vi "output_steps_slower.vi"(7 "# of Samples":i32=7000, 9 "Offset / V":cluster{"X":dbl, "Y":dbl, "Z":dbl}={"X"=0.0, "Y"=0.0, "Z"=0.5}, 10 "Amplitude / V":dbl=0.1 format="%.2g") -> (2 "Output":dbl[][](graph))   [LabVIEW 2018]
panel:
  # "This code is not very adjustable. The number \nof substeps cannot be changed without causing it\nto go haywire and is fixed at 10.\nThe substeps are 300 samples long; 250 as still and \n50 slewing"
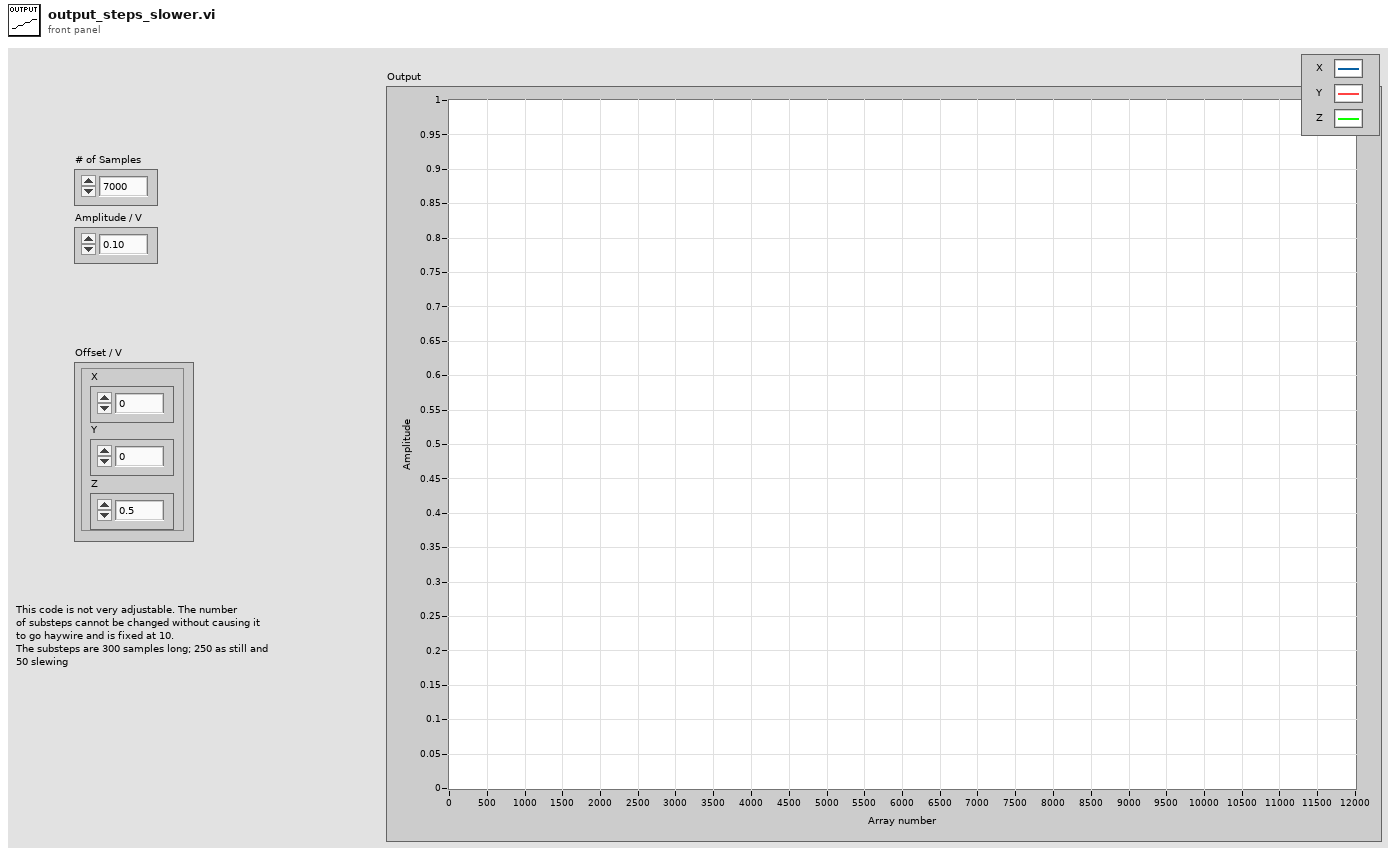
[diagram p1: front panel]
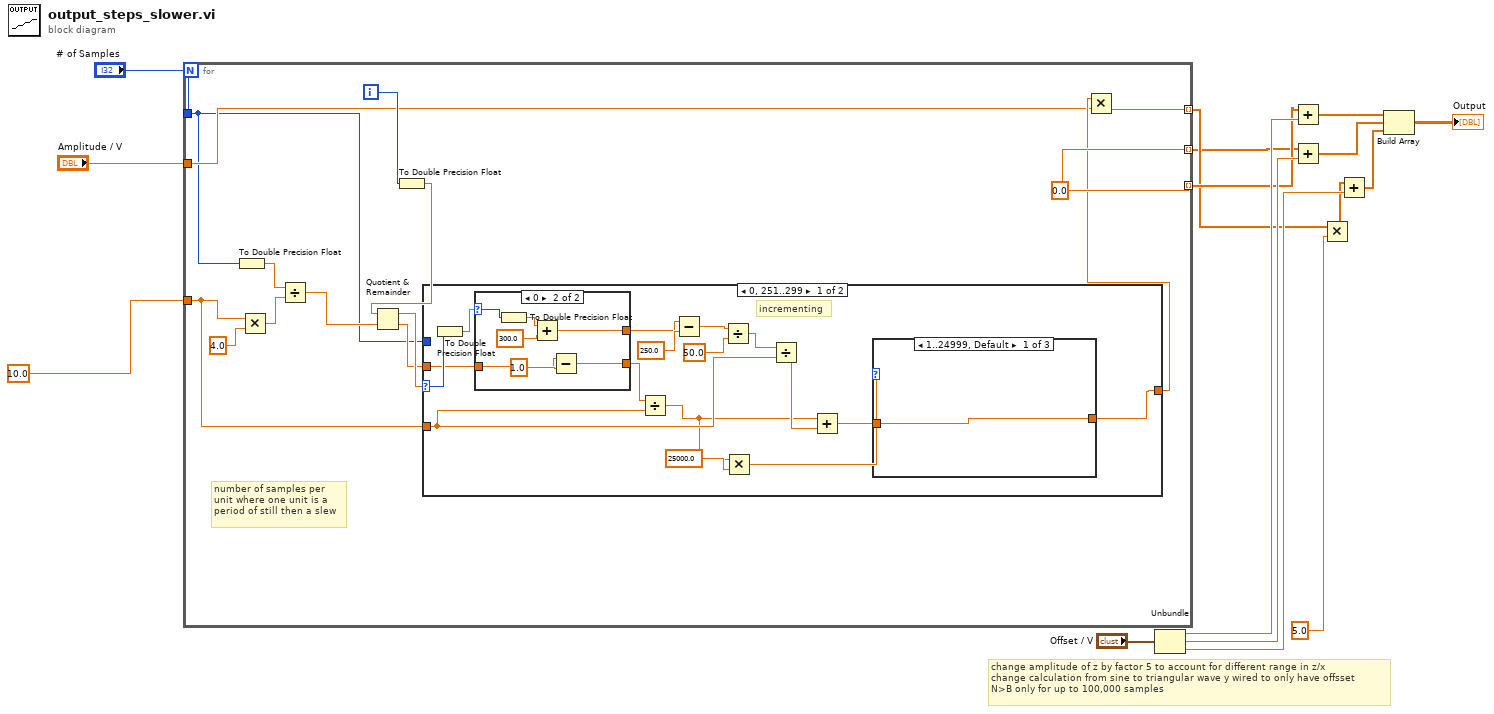
[diagram p0: block diagram]
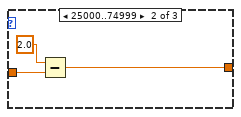
[diagram p3: hidden frame]
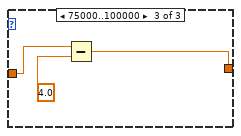
[diagram p4: hidden frame]
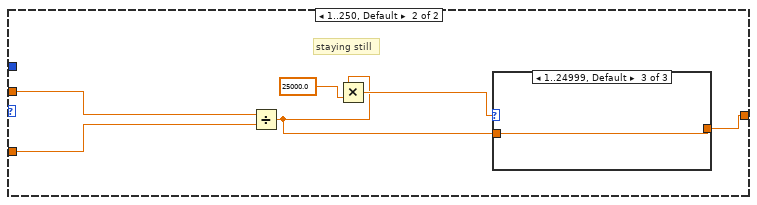
[diagram p5: hidden frame]
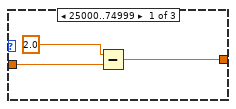
[diagram p6: hidden frame]
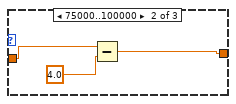
[diagram p7: hidden frame]
diagram:
  # "change amplitude of z by factor 5 to account for different range in z/x\nchange calculation from sine to triangular wave y wired to only have offsset\nN>B only for up to 100,000 samples"
  n1 = for {
    N: "# of Samples" -> [_]
    tunnel: [w30] -> w5 mode=indexing
    tunnel: [w29] -> w2 mode=indexing
    tunnel: "# of Samples" -> [w19]
    tunnel: "Amplitude / V" -> [w20]
    tunnel: [w29] -> w6 mode=indexing
    tunnel: 10.0 ("number of substeps\nin each direction") -> [w17]
    i -> [w22]
    w29 = 0.0
    # "number of samples per \nunit where one unit is a \nperiod of still then a slew"
    n2 = To Double Precision Float(number=w19) -> (double precision float=w27:dbl)
    n3 = Multiply(x=w17, y=4.0) -> (x*y=w18:dbl)
    n4 = Divide(x=w27, y=w18) -> (x/y=w26:dbl)
    n5 = To Double Precision Float(number=w22) -> (double precision float=w21:dbl)
    n6 = Quotient & Remainder(x=w21, y=w26) -> (x-y*floor(x/y)=w25:dbl, floor(x/y)=w24:dbl)
    n7 = case shown="0, 251..299" w25 {
      selector: w25 -> [w35 _]
      tunnel: w24 -> [w32 w68]
      tunnel: w17 -> [w39 w67]
      tunnel: [w46 w64] -> w23
      tunnel: w19 -> [_ _]
      frame 0, 251..299 {
        # "incrementing"
        n8 = To Double Precision Float(number=w35) -> (double precision float=w33:dbl)
        n9 = case shown="0" w33 {
          selector: w33 -> [w48 w53]
          tunnel: [w48 w54] -> w34
          tunnel: w32 -> [w47 w50]
          tunnel: [w47 w49] -> w31
          frame 251..299, Default {
          }
          frame 0 {
            n10 = To Double Precision Float(number=w53) -> (double precision float=w52:dbl)
            n11 = Add(x=w52, y=300.0) -> (x+y=w54:dbl)
            n12 = Subtract(x=w50, y=1.0) -> (x-y=w49:dbl)
          }
        }
        n13 = Divide(x=w31, y=w39) -> (x/y=w37:dbl)
        n14 = Subtract(x=w34, y=250.0) -> (x-y=w43:dbl)
        n15 = Divide(x=w43, y=50.0) -> (x/y=w42:dbl)
        n16 = Multiply(x=w37, y=25000.0) -> (x*y=w36:dbl)
        n17 = Divide(x=w42, y=w39) -> (x/y=w41:dbl)
        n18 = Add(x=w37, y=w41) -> (x+y=w40:dbl)
        n19 = case shown="1..24999, Default" w36 {
          tunnel: w40 -> [w56 w58 w62]
          tunnel: [w56 w57 w60] -> w46
          frame 1..24999, Default {
          }
          frame 25000..74999 {
            n20 = Subtract(x=2.0, y=w58) -> (x-y=w57:dbl)
          }
          frame 75000..100000 {
            n21 = Subtract(x=w62, y=4.0) -> (x-y=w60:dbl)
          }
        }
      }
      frame 1..250, Default {
        # "staying still"
        n22 = Divide(x=w68, y=w67) -> (x/y=w63:dbl)
        n23 = Multiply(x=w63, y=25000.0) -> (x*y=w65:dbl)
        n24 = case shown="1..24999, Default" w65 {
          tunnel: w63 -> [w70 w72 w75]
          tunnel: [w69 w74 w75] -> w64
          frame 25000..74999 {
            n25 = Subtract(x=2.0, y=w70) -> (x-y=w69:dbl)
          }
          frame 75000..100000 {
            n26 = Subtract(x=w72, y=4.0) -> (x-y=w74:dbl)
          }
          frame 1..24999, Default {
          }
        }
      }
    }
    n27 = Multiply(x=w23, y=w20) -> (x*y=w30:dbl)
  }
  n28 = Unbundle("Offset / V") -> ("X"=w13:dbl, "Y"=w12:dbl, "Z"=w11:dbl)
  n29 = Add(x=w6, y=w13) -> (x+y=w10:dbl[])
  n30 = Add(x=w2, y=w12) -> (x+y=w9:dbl[])
  n31 = Multiply(x=w5, y=5.0) -> (x*y=w4:dbl[])
  n32 = Add(x=w4, y=w11) -> (x+y=w8:dbl[])
  n33 = Build Array(w10, w9, w8) -> (→"Output":dbl[][])
